vi "User Table.vi"() -> ()   [LabVIEW 2020, in "User Lib.lvlib"]
uses:
  User Lib.lvlib
  <vilib>/Utility/miscctls.llb/LVRowAndColumnTypeDef.ctl
  <vilib>/addons/database/Connection.llb/DB Tools Open Connec (String).vi
  Database Lib.lvlib
  <vilib>/addons/database/NI_Database_API.lvlib
panel:
  out "Error out 5":errorcluster
  out "Error out 4":errorcluster
  out "Error out 3":errorcluster
  out "Error out 2":errorcluster
  out "Error out":errorcluster
  in  "Cancel":bool
  in  "OK":bool
  in  "Change Pass":bool
  out "data":string[][](array[string])
  in  "Delete":bool
  in  "Update":bool
  in  "New":bool
  out "User Table":string[][](table) caption="Thickness Table"
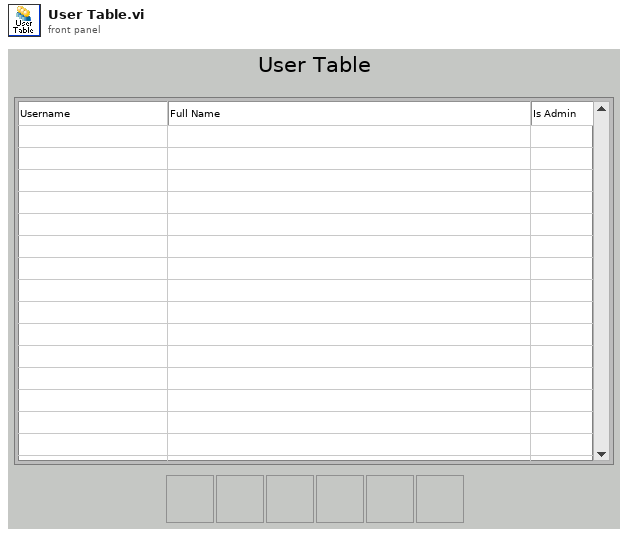
[diagram p1: front panel]
types:
  T1 = typedef "LVRowAndColumnTypeDef.ctl" = cluster{"Row":i32, "Column":i32}
  T2 = cluster{"date/time string":string, "date/time string":string, "code":i32, "date/time string":string, "source":string}
  T3 = typedef "NI_Database_API.lvlib/Conn ObjectReference.ctl" = refnum<k1>
  T4 = cluster{i32, "date/time string":string, "date/time string":string, string}
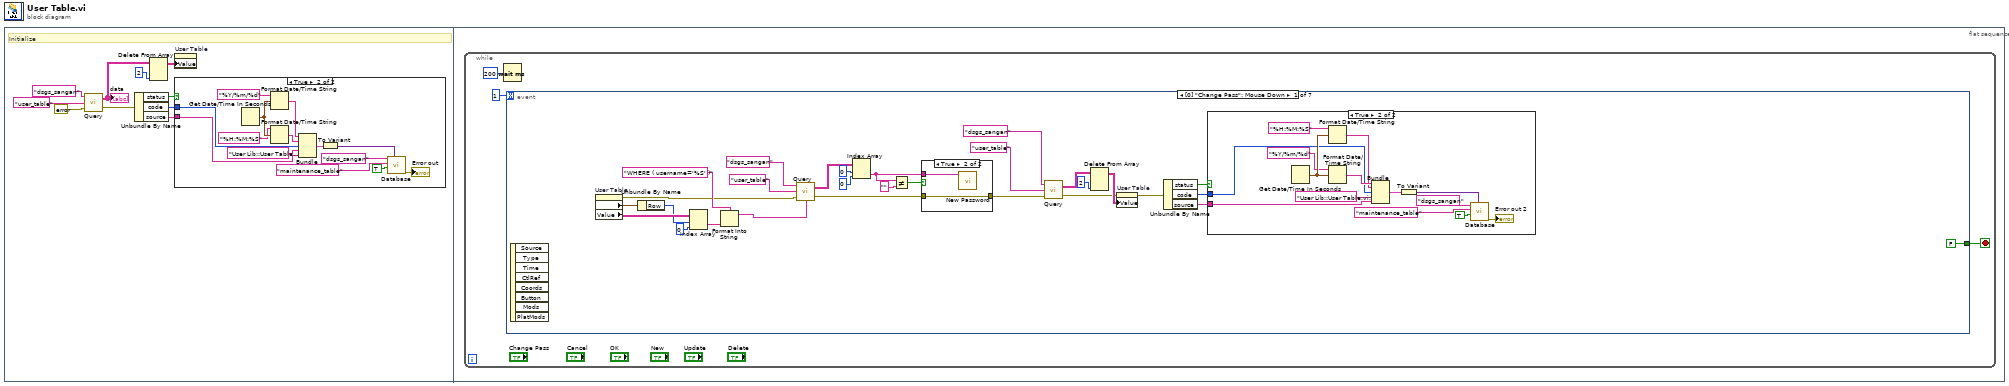
[diagram p0: block diagram]
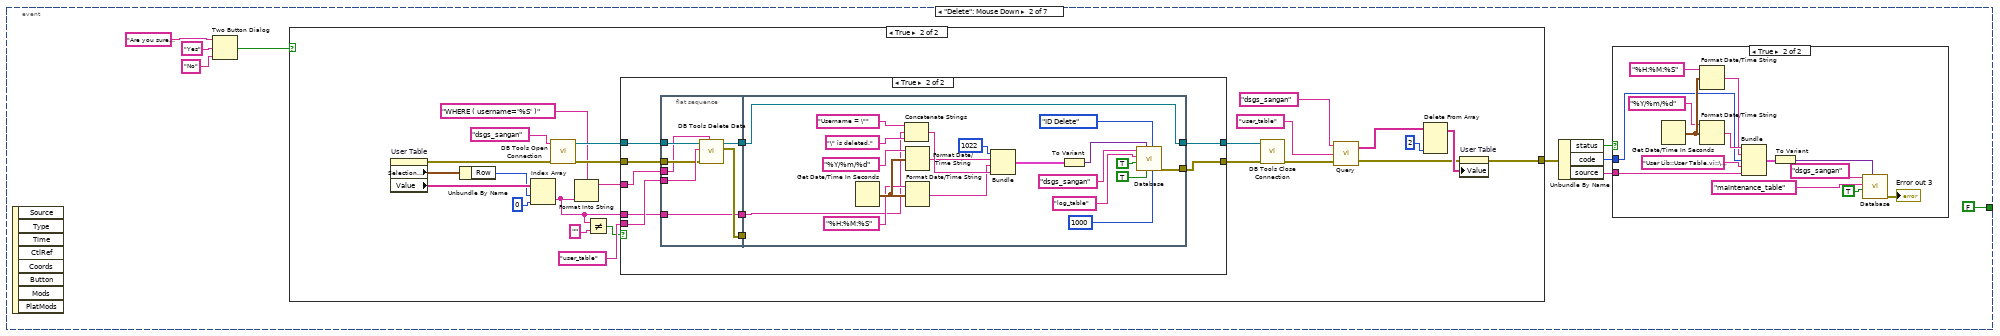
[diagram p5: hidden frame]
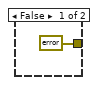
[diagram p7: hidden frame]
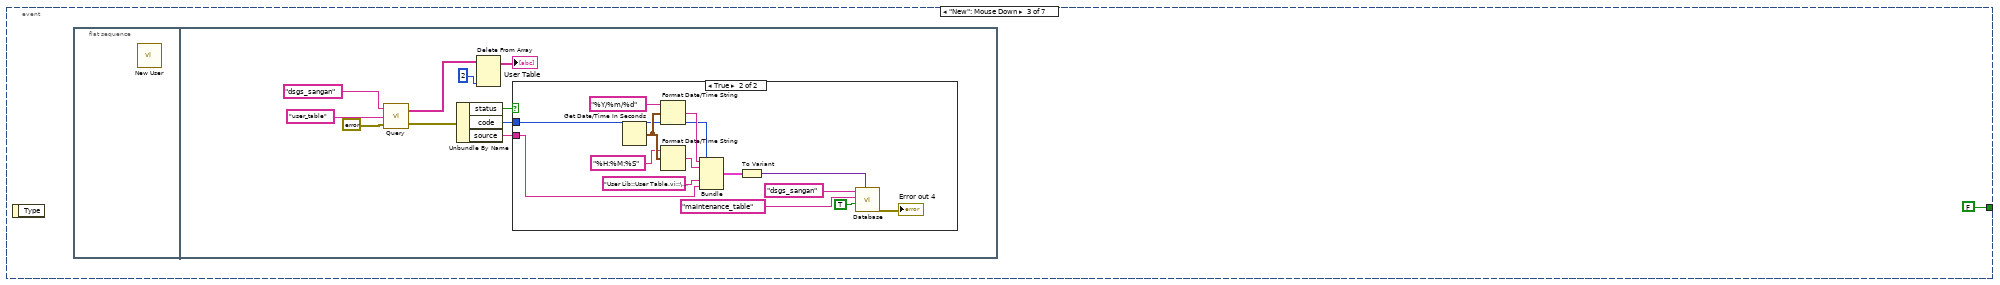
[diagram p9: hidden frame]
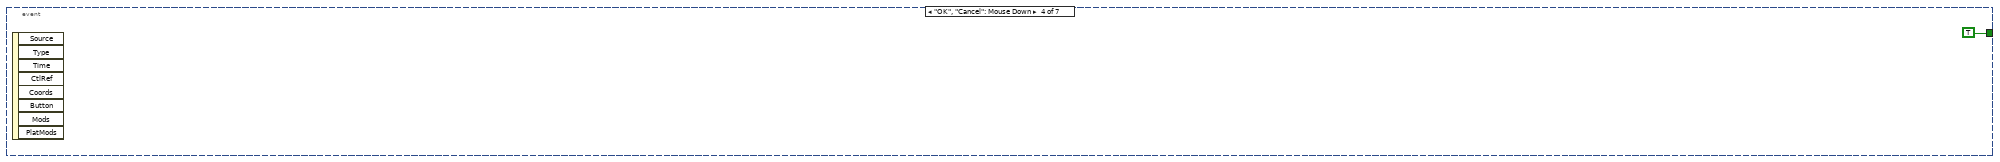
[diagram p11: hidden frame]
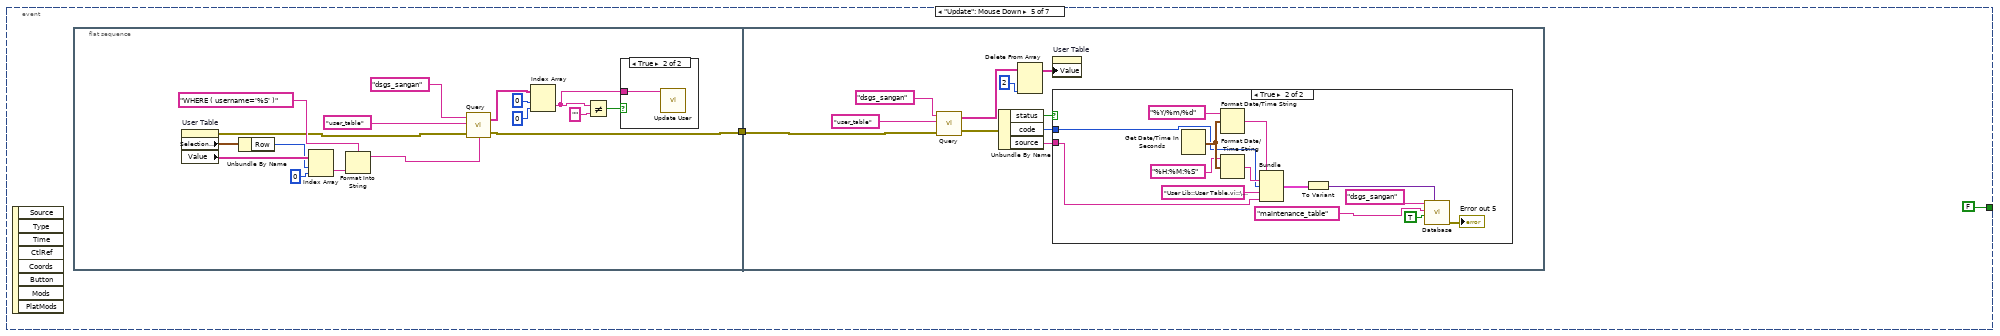
[diagram p12: hidden frame]
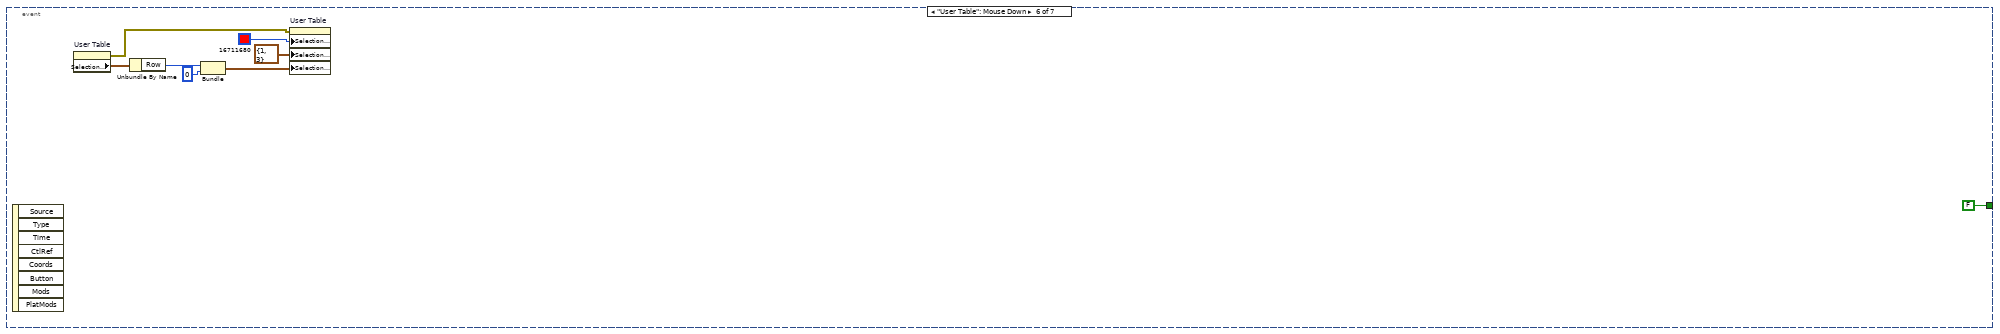
[diagram p15: hidden frame]
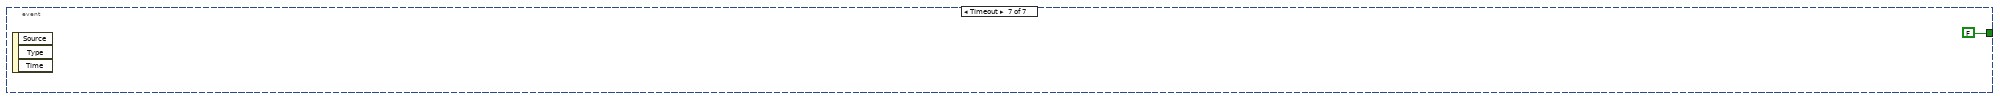
[diagram p16: hidden frame]
diagram:
  n1 = flat-sequence {
    frame #0 {
      # "Initialize"
      n2 = call "Query.vi"("Error in"=errorcluster {"status"=FALSE, "code"=0, "source"=""}, "Table Name"="user_table", "Connection Name"="dsgs_sangan") -> ("Error out"=w1:errorcluster, "data"=w8:string[][])  [unwired: 1 in]
      "data" <- w8
      n3 = Unbundle By Name(w1) -> ("status"=w3:bool, "code"=w4:i32, "source"=w2:string)
      n4 = Delete From Array(array=w8, index (col)=2 ("disabled index (col)")) -> (array with subset deleted=w7:string[][])  [unwired: 2 in, 1 out]
      n5 = property on="User Table" class="Tbl (strict)"("Value"=w7) -> ()  [unwired: 2 in, 2 out]
      n6 = case shown="True" w3 {
        tunnel: w4 -> [_ w19]
        tunnel: w2 -> [_ w17]
        frame False {
        }
        frame True {
          n7 = Get Date/Time In Seconds() -> (seconds since 1Jan1904=w24:timestamp)
          n8 = Format Date/Time String(time format string (%c)="%Y/%m/%d", seconds (now)=w24) -> (date/time string=w21:string)  [unwired: 1 in]
          n9 = Format Date/Time String(time format string (%c)="%H:%M:%S", seconds (now)=w24) -> (date/time string=w20:string)  [unwired: 1 in]
          n10 = Bundle("date/time string"=w21, "date/time string"=w20, "code"=w19, "date/time string"="User Lib::User Table.vi::Initialize", "source"=w17) -> (w16:T2)  [unwired: 1 in]
          n11 = To Variant(anything=w16) -> (Variant=w15:variant)
          n12 = call "Database.vi"("Data"=w15, "Auto Increment ID?"=TRUE, "Table"="maintenance_table", "Connection"="dsgs_sangan") -> ("Error out"=→"Error out":errorcluster)  [unwired: 7 in]
        }
      }
    }
    frame #1 {
      n13 = while {
        stop <- w25 stop-if-true
        n14 = Wait (ms)(milliseconds to wait=u32 200) -> ()  [unwired: 1 out]
        n15 = event shown="[0] \"Change Pass\": Mouse Down" {
          selector: _ -> [_ _ _ _ _ _ _]
          dyn-events: _ -> [_ _ _ _ _ _ _]
          timeout: 1 -> [_ _ _ _ _ _ _]
          tunnel: [FALSE FALSE FALSE TRUE FALSE FALSE FALSE] -> w25
          event "Change Pass": Mouse Down {
            n16 = event-data() -> ()  [unwired: 1 in, 8 out]
            n17 = property on="User Table" class="Tbl (strict)"() -> (error out=w33:errorcluster, "Selection Start"=w55:T1, "Value"=w54:string[][])  [unwired: 2 in, 1 out]
            n18 = Unbundle By Name(w55) -> ("Row"=w53:i32)
            n19 = Index Array(array=w54, index (row)=w53, index (col)=0 ("disabled index (col)")) -> (element=w56:string)
            n20 = Format Into String(format string="WHERE ( username='%S' )" ("condition"), w56) -> (resulting string=w50:string)  [unwired: 2 in, 1 out]
            n21 = call "Query.vi"("Condition"=w50, "Error in"=w33, "Table Name"="user_table", "Connection Name"="dsgs_sangan") -> ("Error out"=w51:errorcluster, "data"=w49:string[][])
            n22 = Index Array(array=w49, index (row)=0, index (col)=0 ("disabled index (col)")) -> (element=w48:string)
            n23 = Not Equal?(x=w48, y="") -> (x != y?=w47:bool)
            n24 = case shown="True" w47 {
              tunnel: [w71 w72] -> w52
              tunnel: w51 -> [w71 w72]
              tunnel: w48 -> [_ w73]
              frame False {
              }
              frame True {
                n25 = call "New Password.vi"("Username"=w73) -> ()  [unwired: 11 in]
              }
            }
            n26 = call "Query.vi"("Error in"=w52, "Table Name"="user_table", "Connection Name"="dsgs_sangan") -> ("Error out"=w32:errorcluster, "data"=w46:string[][])  [unwired: 1 in]
            n27 = Delete From Array(array=w46, index (col)=2 ("disabled index (col)")) -> (array with subset deleted=w45:string[][])  [unwired: 2 in, 1 out]
            n28 = property on="User Table" class="Tbl (strict)"(error in=w32, "Value"=w45) -> (error out=w28:errorcluster)  [unwired: 1 in, 1 out]
            n29 = Unbundle By Name(w28) -> ("status"=w30:bool, "code"=w31:i32, "source"=w29:string)
            n30 = case shown="True" w30 {
              tunnel: w31 -> [_ w65]
              tunnel: w29 -> [_ w63]
              frame False {
              }
              frame True {
                n31 = Get Date/Time In Seconds() -> (seconds since 1Jan1904=w70:timestamp)
                n32 = Format Date/Time String(time format string (%c)="%H:%M:%S", seconds (now)=w70) -> (date/time string=w66:string)  [unwired: 1 in]
                n33 = Format Date/Time String(time format string (%c)="%Y/%m/%d", seconds (now)=w70) -> (date/time string=w67:string)  [unwired: 1 in]
                n34 = Bundle("date/time string"=w67, "date/time string"=w66, "code"=w65, "date/time string"="User Lib::User Table.vi::\"Change Pass\" case", "source"=w63) -> (w62:T2)  [unwired: 1 in]
                n35 = To Variant(anything=w62) -> (Variant=w61:variant)
                n36 = call "Database.vi"("Data"=w61, "Auto Increment ID?"=TRUE, "Table"="maintenance_table", "Connection"="dsgs_sangan") -> ("Error out"=→"Error out 2":errorcluster)  [unwired: 7 in]
              }
            }
          }
          event "Delete": Mouse Down {
            n37 = event-data() -> ()  [unwired: 1 in, 8 out]
            n38 = Two Button Dialog(message="Are you sure to delete this user?", 1:"No" ("F button name (\"Cancel\")"), 2:"Yes" ("T button name (\"OK\")")) -> (T button?=w82:bool)
            n39 = case shown="True" w82 {
              tunnel: [errorcluster {"status"=FALSE, "code"=0, "source"=""} ("error out") w98] -> w74
              frame False {
              }
              frame True {
                n40 = property on="User Table" class="Tbl (strict)"() -> (error out=w100:errorcluster, "Selection Start"=w121:T1, "Value"=w116:string[][])  [unwired: 2 in, 1 out]
                n41 = Unbundle By Name(w121) -> ("Row"=w115:i32)
                n42 = Index Array(array=w116, index (row)=w115, index (col)=0 ("disabled index (col)")) -> (element=w101:string)
                n43 = call-poly <vilib>:"DB Tools Open Connection.vi"("error in (no error)"=w100, "connection information"="dsgs_sangan") -> ("error out"=w117:errorcluster, "connection reference"=w119:T3)  [unwired: 6 in]
                n44 = Format Into String(format string="WHERE ( username='%S' )" ("condition"), w101) -> (resulting string=w108:string)  [unwired: 2 in, 1 out]
                n45 = Not Equal?(x=w101, y="") -> (x != y?=w106:bool)
                n46 = case shown="True" w106 {
                  tunnel: w119 -> [w123 w133]
                  tunnel: "user_table" ("table") -> [_ w132]
                  tunnel: w117 -> [w122 w131]
                  tunnel: [w123 w130] -> w113
                  tunnel: [w122 w129] -> w112
                  tunnel: w108 -> [_ w128]
                  tunnel: w101 -> [_ w125]
                  frame False {
                  }
                  frame True {
                    n47 = flat-sequence {
                      tunnel: w133 -> [w140]
                      tunnel: w132 -> [w139]
                      tunnel: w131 -> [w138]
                      tunnel: w128 -> [w135]
                      tunnel: [w137] -> w127
                      tunnel: [w136] -> w126
                      tunnel: w125 -> [w134]
                      tunnel: [w134] -> w124
                      tunnel: [w145] -> w129
                      tunnel: [w160] -> w130
                      tunnel: w127 -> [w160]
                      tunnel: w126 -> [_]
                      tunnel: w124 -> [w144]
                      frame #0 {
                        n48 = call <vilib>:"DB Tools Delete Data.vi"("condition"=w135, "error in (no error)"=w138, "table"=w139, "connection reference"=w140) -> ("error out"=w136:errorcluster, "connection reference out"=w137:T3)  [unwired: 6 in]
                      }
                      frame #1 {
                        n49 = Get Date/Time In Seconds() -> (seconds since 1Jan1904=w158:timestamp)
                        n50 = Concatenate Strings("Username = \"" ("string"), w144, "\" is deleted." ("string")) -> (w159:string)
                        n51 = Format Date/Time String(time format string (%c)="%Y/%m/%d", seconds (now)=w158) -> (date/time string=w157:string)  [unwired: 1 in]
                        n52 = Format Date/Time String(time format string (%c)="%H:%M:%S", seconds (now)=w158) -> (date/time string=w156:string)  [unwired: 1 in]
                        n53 = Bundle(1022, "date/time string"=w157, "date/time string"=w156, w159) -> (w155:T4)  [unwired: 1 in]
                        n54 = To Variant(anything=w155) -> (Variant=w154:variant)
                        n55 = call "Database.vi"("Maximum Row"=1000, "Enum"=enum16{"ID Delete", "Time Delete"}."ID Delete", "Delete row?"=TRUE, "Data"=w154, "Auto Increment ID?"=TRUE, "Table"="log_table" ("table"), "Connection"="dsgs_sangan" ("table")) -> ("Error out"=w145:errorcluster)  [unwired: 4 in]
                      }
                    }
                  }
                }
                n56 = call <vilib>:"DB Tools Close Connection.vi"("error in (no error)"=w112, "connection reference"=w113) -> ("error out"=w109:errorcluster)  [unwired: 5 in]
                n57 = call "Query.vi"("Error in"=w109, "Table Name"="user_table", "Connection Name"="dsgs_sangan") -> ("Error out"=w99:errorcluster, "data"=w103:string[][])  [unwired: 1 in]
                n58 = Delete From Array(array=w103, index (col)=2 ("disabled index (col)")) -> (array with subset deleted=w102:string[][])  [unwired: 2 in, 1 out]
                n59 = property on="User Table" class="Tbl (strict)"(error in=w99, "Value"=w102) -> (error out=w98:errorcluster)  [unwired: 1 in, 1 out]
              }
            }
            n60 = Unbundle By Name(w74) -> ("status"=w76:bool, "code"=w77:i32, "source"=w75:string)
            n61 = case shown="True" w76 {
              tunnel: w77 -> [_ w91]
              tunnel: w75 -> [_ w89]
              frame False {
              }
              frame True {
                n62 = Get Date/Time In Seconds() -> (seconds since 1Jan1904=w96:timestamp)
                n63 = Format Date/Time String(time format string (%c)="%H:%M:%S", seconds (now)=w96) -> (date/time string=w92:string)  [unwired: 1 in]
                n64 = Format Date/Time String(time format string (%c)="%Y/%m/%d", seconds (now)=w96) -> (date/time string=w93:string)  [unwired: 1 in]
                n65 = Bundle("date/time string"=w93, "date/time string"=w92, "code"=w91, "date/time string"="User Lib::User Table.vi::\"Delete\" case", "source"=w89) -> (w88:T2)  [unwired: 1 in]
                n66 = To Variant(anything=w88) -> (Variant=w87:variant)
                n67 = call "Database.vi"("Data"=w87, "Auto Increment ID?"=TRUE, "Table"="maintenance_table", "Connection"="dsgs_sangan") -> ("Error out"=→"Error out 3":errorcluster)  [unwired: 7 in]
              }
            }
          }
          event "New": Mouse Down {
            n68 = event-data() -> ()  [unwired: 1 in, 1 out]
            n69 = flat-sequence {
              frame #0 {
                n70 = call "New User.vi"() -> ()  [unwired: 12 in]
              }
              frame #1 {
                n71 = call "Query.vi"("Error in"=errorcluster {"status"=FALSE, "code"=0, "source"=""}, "Table Name"="user_table", "Connection Name"="dsgs_sangan") -> ("Error out"=w163:errorcluster, "data"=w169:string[][])  [unwired: 1 in]
                n72 = Unbundle By Name(w163) -> ("status"=w165:bool, "code"=w166:i32, "source"=w164:string)
                n73 = Delete From Array(array=w169, index (col)=2 ("disabled index (col)")) -> (array with subset deleted=→"User Table":string[][])  [unwired: 2 in, 1 out]
                n74 = case shown="True" w165 {
                  tunnel: w166 -> [_ w180]
                  tunnel: w164 -> [_ w178]
                  frame False {
                  }
                  frame True {
                    n75 = Get Date/Time In Seconds() -> (seconds since 1Jan1904=w185:timestamp)
                    n76 = Format Date/Time String(time format string (%c)="%Y/%m/%d", seconds (now)=w185) -> (date/time string=w182:string)  [unwired: 1 in]
                    n77 = Format Date/Time String(time format string (%c)="%H:%M:%S", seconds (now)=w185) -> (date/time string=w181:string)  [unwired: 1 in]
                    n78 = Bundle("date/time string"=w182, "date/time string"=w181, "code"=w180, "date/time string"="User Lib::User Table.vi::\"New\" case", "source"=w178) -> (w177:T2)  [unwired: 1 in]
                    n79 = To Variant(anything=w177) -> (Variant=w176:variant)
                    n80 = call "Database.vi"("Data"=w176, "Auto Increment ID?"=TRUE, "Table"="maintenance_table", "Connection"="dsgs_sangan") -> ("Error out"=→"Error out 4":errorcluster)  [unwired: 7 in]
                  }
                }
              }
            }
          }
          event "OK", "Cancel": Mouse Down {
            n81 = event-data() -> ()  [unwired: 1 in, 8 out]
          }
          event "Update": Mouse Down {
            n82 = event-data() -> ()  [unwired: 1 in, 8 out]
            n83 = flat-sequence {
              tunnel: [w190] -> w187
              tunnel: w187 -> [w211]
              frame #0 {
                n84 = property on="User Table" class="Tbl (strict)"() -> (error out=w189:errorcluster, "Selection Start"=w205:T1, "Value"=w204:string[][])  [unwired: 2 in, 1 out]
                n85 = Unbundle By Name(w205) -> ("Row"=w203:i32)
                n86 = Index Array(array=w204, index (row)=w203, index (col)=0 ("disabled index (col)")) -> (element=w202:string)
                n87 = Format Into String(format string="WHERE ( username='%S' )" ("condition"), w202) -> (resulting string=w197:string)  [unwired: 2 in, 1 out]
                n88 = call "Query.vi"("Condition"=w197, "Error in"=w189, "Table Name"="user_table", "Connection Name"="dsgs_sangan") -> ("Error out"=w190:errorcluster, "data"=w196:string[][])
                n89 = Index Array(array=w196, index (row)=0, index (col)=0 ("disabled index (col)")) -> (element=w193:string)
                n90 = Not Equal?(x=w193, y="") -> (x != y?=w192:bool)
                n91 = case shown="True" w192 {
                  tunnel: w193 -> [_ w206]
                  frame False {
                  }
                  frame True {
                    n92 = call "Update User.vi"("Username"=w206) -> ()  [unwired: 11 in]
                  }
                }
              }
              frame #1 {
                n93 = call "Query.vi"("Error in"=w211, "Table Name"="user_table", "Connection Name"="dsgs_sangan") -> ("Error out"=w207:errorcluster, "data"=w215:string[][])  [unwired: 1 in]
                n94 = Unbundle By Name(w207) -> ("status"=w209:bool, "code"=w210:i32, "source"=w208:string)
                n95 = Delete From Array(array=w215, index (col)=2 ("disabled index (col)")) -> (array with subset deleted=w216:string[][])  [unwired: 2 in, 1 out]
                n96 = property on="User Table" class="Tbl (strict)"("Value"=w216) -> ()  [unwired: 2 in, 2 out]
                n97 = case shown="True" w209 {
                  tunnel: w210 -> [_ w225]
                  tunnel: w208 -> [_ w223]
                  frame False {
                  }
                  frame True {
                    n98 = Get Date/Time In Seconds() -> (seconds since 1Jan1904=w230:timestamp)
                    n99 = Format Date/Time String(time format string (%c)="%Y/%m/%d", seconds (now)=w230) -> (date/time string=w227:string)  [unwired: 1 in]
                    n100 = Format Date/Time String(time format string (%c)="%H:%M:%S", seconds (now)=w230) -> (date/time string=w226:string)  [unwired: 1 in]
                    n101 = Bundle("date/time string"=w227, "date/time string"=w226, "code"=w225, "date/time string"="User Lib::User Table.vi::\"Update\" case", "source"=w223) -> (w222:T2)  [unwired: 1 in]
                    n102 = To Variant(anything=w222) -> (Variant=w221:variant)
                    n103 = call "Database.vi"("Data"=w221, "Auto Increment ID?"=TRUE, "Table"="maintenance_table", "Connection"="dsgs_sangan") -> ("Error out"=→"Error out 5":errorcluster)  [unwired: 7 in]
                  }
                }
              }
            }
          }
          event "User Table": Mouse Down {
            n104 = event-data() -> ()  [unwired: 1 in, 8 out]
            n105 = property on="User Table" class="Tbl (strict)"() -> (error out=w231:errorcluster, "Selection Start"=w235:T1)  [unwired: 2 in, 1 out]
            n106 = Unbundle By Name(w235) -> ("Row"=w236:i32)
            n107 = Bundle("Row"=w236, "Row"=0) -> (w238:cluster{"Row":i32, "Row":i32})  [unwired: 1 in]
            n108 = property on="User Table" class="Tbl (strict)"(error in=w231, "Selection Color"=u32 16711680, "Selection Size"=T1 {"Row"=1, "Column"=3}, "Selection Start"=w238) -> ()  [unwired: 1 in, 2 out]
          }
          event Timeout {
            n109 = event-data() -> ()  [unwired: 1 in, 3 out]
          }
        }
      }
    }
  }
